vi "FA OffsetForces View.vi"(11 "Model in":refnum<class "Model.lvclass">) -> ()   [LabVIEW 2016, in "M1M3SupportEUI_Views.lvlib"]
uses:
  M1M3SupportEUI_Views.lvlib
  Model/Model.lvclass
  M1M3 Support Events/M1M3 Support Events.lvclass/M1M3 Support Events.ctl
  SALLV_m1m3/DataTypes/command_ApplyOffsetForces.ctl
  SALLV_m1m3/DataTypes/command_ClearOffsetForces.ctl
  M1M3 Support Events/M1M3 Support Events.lvclass
  EUI Events/EUI Events.lvclass
  SALLV_m1m3/SALLV_m1m3.lvlib
panel:
  in  "Z441":sgl
  in  "Z440":sgl
  in  "Z443":sgl
  in  "Z442":sgl
  in  "Z401":sgl
  in  "Z431":sgl
  in  "Z430":sgl
  in  "Z439":sgl
  in  "Z438":sgl
  in  "Z437":sgl
  in  "Z436":sgl
  in  "Z435":sgl
  in  "Z434":sgl
  in  "Z433":sgl
  in  "Z432":sgl
  in  "Z421":sgl
  in  "Z420":sgl
  in  "Z429":sgl
  in  "Z428":sgl
  in  "Z427":sgl
  in  "Z426":sgl
  in  "Z425":sgl
  in  "Z424":sgl
  in  "Z423":sgl
  in  "Z422":sgl
  in  "Z411":sgl
  in  "Z410":sgl
  in  "Z419":sgl
  in  "Z418":sgl
  in  "Z417":sgl
  in  "Z416":sgl
  in  "Z415":sgl
  in  "Z414":sgl
  in  "Z413":sgl
  in  "Z412":sgl
  in  "Z409":sgl
  in  "Z408":sgl
  in  "Z407":sgl
  in  "Z406":sgl
  in  "Z405":sgl
  in  "Z404":sgl
  in  "Z403":sgl
  in  "Z402":sgl
  in  "Z341":sgl
  in  "Z340":sgl
  in  "Z343":sgl
  in  "Z342":sgl
  in  "Z301":sgl
  in  "Z331":sgl
  in  "Z330":sgl
  in  "Z339":sgl
  in  "Z338":sgl
  in  "Z337":sgl
  in  "Z336":sgl
  in  "Z335":sgl
  in  "Z334":sgl
  in  "Z333":sgl
  in  "Z332":sgl
  in  "Z321":sgl
  in  "Z320":sgl
  in  "Z329":sgl
  in  "Z328":sgl
  in  "Z327":sgl
  in  "Z326":sgl
  in  "Z325":sgl
  in  "Z324":sgl
  in  "Z323":sgl
  in  "Z322":sgl
  in  "Z311":sgl
  in  "Z310":sgl
  in  "Z319":sgl
  in  "Z318":sgl
  in  "Z317":sgl
  in  "Z316":sgl
  in  "Z315":sgl
  in  "Z314":sgl
  in  "Z313":sgl
  in  "Z312":sgl
  in  "Z309":sgl
  in  "Z308":sgl
  in  "Z307":sgl
  in  "Z306":sgl
  in  "Z305":sgl
  in  "Z304":sgl
  in  "Z303":sgl
  in  "Z302":sgl
  in  "Z241":sgl
  in  "Z240":sgl
  in  "Z243":sgl
  in  "Z242":sgl
  in  "Z201":sgl
  in  "Z231":sgl
  in  "Z230":sgl
  in  "Z239":sgl
  in  "Z238":sgl
  in  "Z237":sgl
  in  "Z236":sgl
  in  "Z235":sgl
  in  "Z234":sgl
  in  "Z233":sgl
  in  "Z232":sgl
  in  "Z221":sgl
  in  "Z220":sgl
  in  "Z229":sgl
  in  "Z228":sgl
  in  "Z227":sgl
  in  "Z226":sgl
  in  "Z225":sgl
  in  "Z224":sgl
  in  "Z223":sgl
  in  "Z222":sgl
  in  "Z211":sgl
  in  "Z210":sgl
  in  "Z219":sgl
  in  "Z218":sgl
  in  "Z217":sgl
  in  "Z216":sgl
  in  "Z215":sgl
  in  "Z214":sgl
  in  "Z213":sgl
  in  "Z212":sgl
  in  "Z209":sgl
  in  "Z208":sgl
  in  "Z207":sgl
  in  "Z206":sgl
  in  "Z205":sgl
  in  "Z204":sgl
  in  "Z203":sgl
  in  "Z202":sgl
  in  "Y430":sgl
  in  "Y438":sgl
  in  "Y437":sgl
  in  "Y434":sgl
  in  "Y433":sgl
  in  "Y432":sgl
  in  "Y421":sgl
  in  "Y420":sgl
  in  "Y429":sgl
  in  "Y427":sgl
  in  "Y424":sgl
  in  "Y423":sgl
  in  "Y422":sgl
  in  "Y411":sgl
  in  "Y410":sgl
  in  "Y418":sgl
  in  "Y417":sgl
  in  "Y416":sgl
  in  "Y415":sgl
  in  "Y414":sgl
  in  "Y409":sgl
  in  "Y408":sgl
  in  "Y230":sgl
  in  "Y238":sgl
  in  "Y237":sgl
  in  "Y234":sgl
  in  "Y233":sgl
  in  "Y232":sgl
  in  "Y221":sgl
  in  "Y220":sgl
  in  "Y229":sgl
  in  "Y227":sgl
  in  "Y224":sgl
  in  "Y223":sgl
  in  "Y222":sgl
  in  "Y211":sgl
  in  "Y210":sgl
  in  "Y218":sgl
  in  "Y217":sgl
  in  "Y216":sgl
  in  "Y215":sgl
  in  "Y214":sgl
  in  "Y209":sgl
  in  "Y208":sgl
  in  "Y330":sgl
  in  "Y338":sgl
  in  "Y337":sgl
  in  "Y334":sgl
  in  "Y333":sgl
  in  "Y332":sgl
  in  "Y321":sgl
  in  "Y320":sgl
  in  "Y329":sgl
  in  "Y327":sgl
  in  "Y326":sgl
  in  "Y324":sgl
  in  "Y323":sgl
  in  "Y322":sgl
  in  "Y311":sgl
  in  "Y310":sgl
  in  "Y318":sgl
  in  "Y317":sgl
  in  "Y316":sgl
  in  "Y315":sgl
  in  "Y314":sgl
  in  "Y313":sgl
  in  "Y309":sgl
  in  "Y308":sgl
  in  "Y305":sgl
  in  "Y304":sgl
  in  "Y303":sgl
  in  "Y302":sgl
  in  "Z141":sgl
  in  "Z140":sgl
  in  "Z143":sgl
  in  "Z142":sgl
  in  "Z101":sgl
  in  "Z131":sgl
  in  "Z130":sgl
  in  "Z139":sgl
  in  "Z138":sgl
  in  "Z137":sgl
  in  "Z136":sgl
  in  "Z135":sgl
  in  "Z134":sgl
  in  "Z133":sgl
  in  "Z132":sgl
  in  "Z121":sgl
  in  "Z120":sgl
  in  "Z129":sgl
  in  "Z128":sgl
  in  "Z127":sgl
  in  "Z126":sgl
  in  "Z125":sgl
  in  "Z124":sgl
  in  "Z123":sgl
  in  "Z122":sgl
  in  "Z111":sgl
  in  "Z110":sgl
  in  "Z119":sgl
  in  "Z118":sgl
  in  "Z117":sgl
  in  "Z116":sgl
  in  "Z115":sgl
  in  "Z114":sgl
  in  "Z113":sgl
  in  "Z112":sgl
  in  "Z109":sgl
  in  "Z108":sgl
  in  "Z107":sgl
  in  "Z106":sgl
  in  "Z105":sgl
  in  "Z104":sgl
  in  "Z103":sgl
  in  "Z102":sgl
  in  "Y130":sgl
  in  "Y138":sgl
  in  "Y137":sgl
  in  "Y134":sgl
  in  "Y133":sgl
  in  "Y132":sgl
  in  "Y121":sgl
  in  "Y120":sgl
  in  "Y129":sgl
  in  "Y127":sgl
  in  "Y126":sgl
  in  "Y124":sgl
  in  "Y123":sgl
  in  "Y122":sgl
  in  "Y111":sgl
  in  "Y110":sgl
  in  "Y118":sgl
  in  "Y117":sgl
  in  "Y116":sgl
  in  "Y115":sgl
  in  "Y114":sgl
  in  "Y113":sgl
  in  "Y109":sgl
  in  "Y108":sgl
  in  "Y105":sgl
  in  "Y104":sgl
  in  "Y103":sgl
  in  "ClearForcesButton":bool
  in  "ApplyForcesButton":bool
  in  "Y102":sgl
  in  "X435":sgl
  in  "X428":sgl
  in  "X412":sgl
  in  "X335":sgl
  in  "X328":sgl
  in  "X312":sgl
  in  "X235":sgl
  in  "X228":sgl
  in  "X212":sgl
  in  "X135":sgl
  in  "X128":sgl
  in  "X112":sgl
  # "Force Actuator\nApply Forces"
  # "Y"
  # "Z"
  # "0"
  # "1"
  # "2"
  # "3"
  # "4"
  # "5"
  # "6"
  # "7"
  # "8"
  # "9"
  # "0"
  # "1"
  # "2"
  # "3"
  # "4"
  # "5"
  # "6"
  # "7"
  # "8"
  # "9"
  # "100"
  # "100"
  # "X"
  # "110"
  # "110"
  # "112"
  # "120"
  # "120"
  # "128"
  # "130"
  # "130"
  # "135"
  # "140"
  # "140"
  # "212"
  # "200"
  # "200"
  # "228"
  # "210"
  # "210"
  # "235"
  # "220"
  # "220"
  # "312"
  # "230"
  # "230"
  # "328"
  # "240"
  # "240"
  # "335"
  # "300"
  # "300"
  # "412"
  # "310"
  # "310"
  # "428"
  # "320"
  # "320"
  # "435"
  # "330"
  # "330"
  # "340"
  # "340"
  # "400"
  # "400"
  # "410"
  # "410"
  # "420"
  # "420"
  # "430"
  # "430"
  # "440"
  # "440"
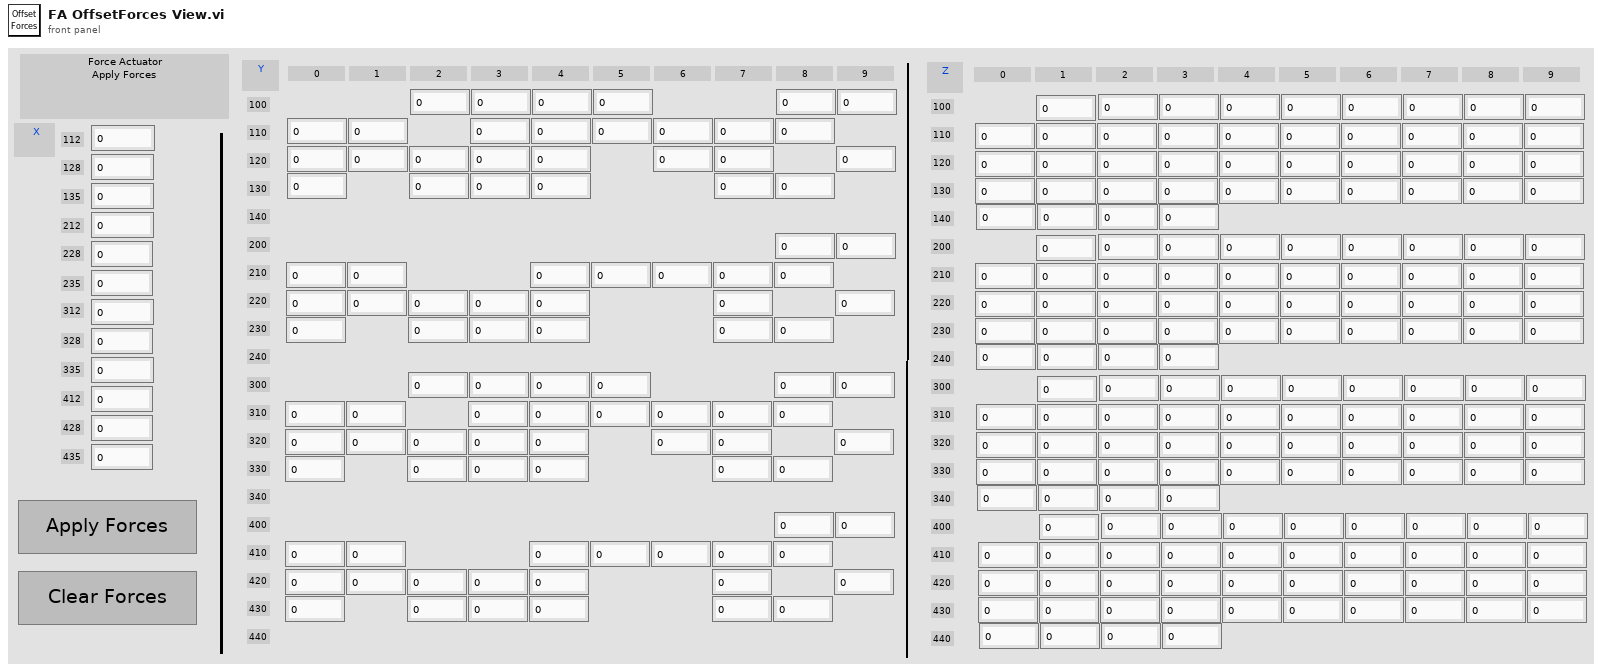
[diagram p1: front panel]
types:
  T1 = typedef "M1M3SupportEUI_TypeDefs.lvlib/M1M3 Support Events.ctl" = cluster{"Inclinometer  Data":refnum<user-event>, "IMS Data":refnum<user-event>, "FA Status":refnum<user-event>, "SAL Connected":refnum<user-event>, "Accelerometer Data":refnum<user-event>, "OuterLoop Data":refnum<user-event>, "ErrorCode Event":refnum<user-event>, "InterlockStatus Event":refnum<user-event>, "InterlockWarning Event":refnum<user-event>, "Gyro Data":refnum<user-event>, "HP Actuator Info Event":refnum<user-event>, " FA Info Event":refnum<user-event>, "HP Monitor Info Event":refnum<user-event>, "FA Data":refnum<user-event>, "HP Actuator data":refnum<user-event>, "HP Monitor data":refnum<user-event>, "Air Supply Status Event":refnum<user-event>, "Air Supply Warning Event":refnum<user-event>, "Power Data":refnum<user-event>, "PID Data":refnum<user-event>, "PID Info Event":refnum<user-event>, "Power Status Event":refnum<user-event>, "Power Supply Status Event":refnum<user-event>, "Power Warning Event":refnum<user-event>, "Summary State Event":refnum<user-event>, "Detailed State Event":refnum<user-event>}
  T2 = enum16{"", "DetailedState_DetailedStates_DisabledState", "DetailedState_DetailedStates_EnabledState", "DetailedState_DetailedStates_FaultState", "DetailedState_DetailedStates_OfflineState", "DetailedState_DetailedStates_StandbyState", "DetailedState_DetailedStates_ParkedState", "DetailedState_DetailedStates_RaisingState", "DetailedState_DetailedStates_ActiveState", "DetailedState_DetailedStates_LoweringState", "DetailedState_DetailedStates_EngineeringState", "DetailedState_DetailedStates_ParkedEngineeringState", "DetailedState_DetailedStates_RaisingEngineeringState", "DetailedState_DetailedStates_ActiveEngineeringState", "DetailedState_DetailedStates_LoweringEngineeringState", "DetailedState_DetailedStates_LoweringFaultState", "DetailedState_DetailedStates_ProfileHardpointCorrectionState"}
  T3 = typedef "SALLV_m1m3.lvlib/command_ApplyOffsetForces.ctl" = cluster{"XForces[12]":sgl[], "YForces[100]":sgl[], "ZForces[156]":sgl[]}
  T4 = typedef "SALLV_m1m3.lvlib/command_ClearOffsetForces.ctl" = cluster{"ClearOffsetForces":bool}
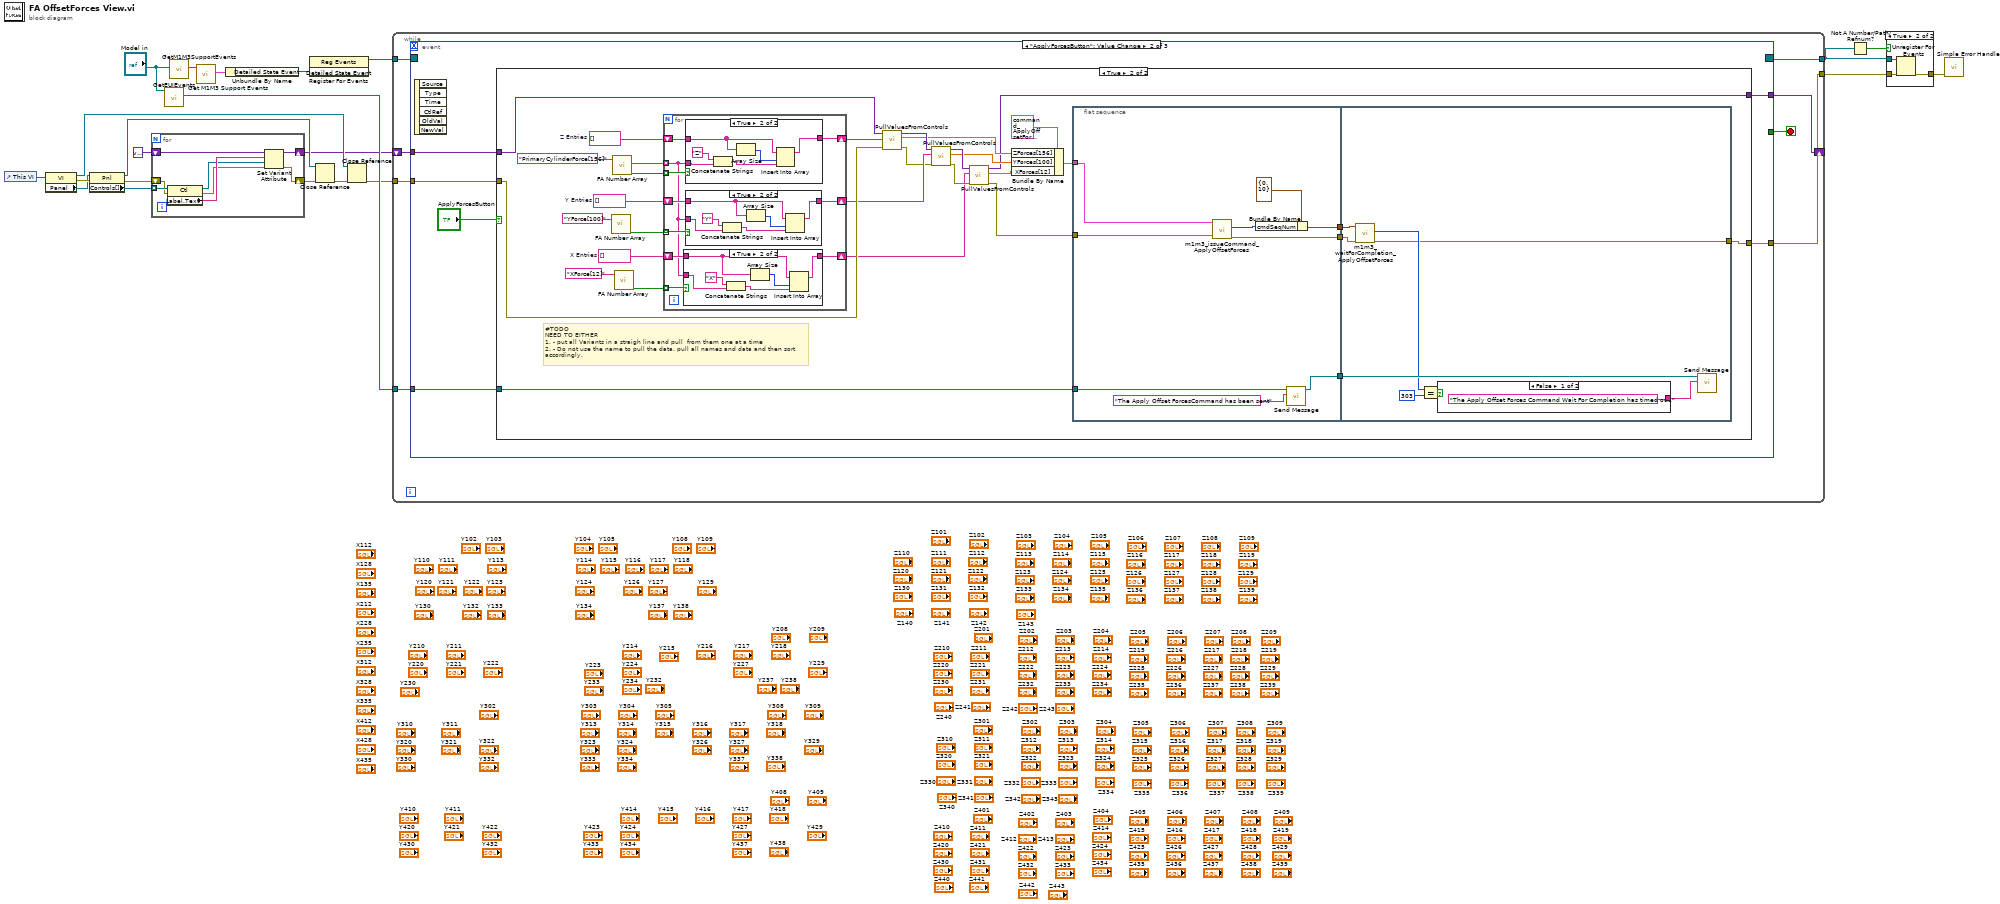
[diagram p0: block diagram]
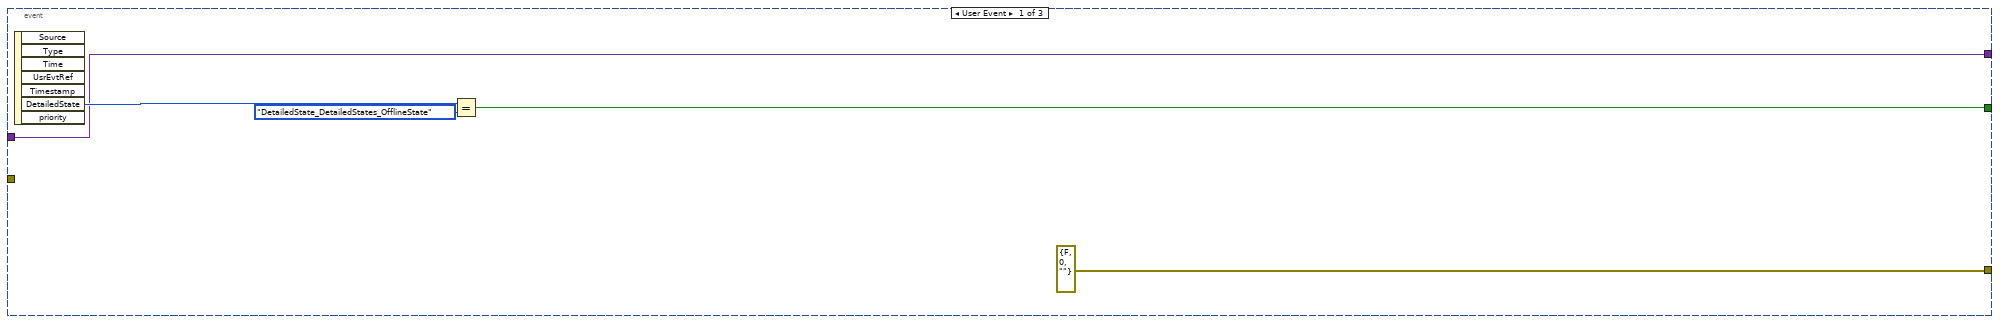
[diagram p2: hidden frame]
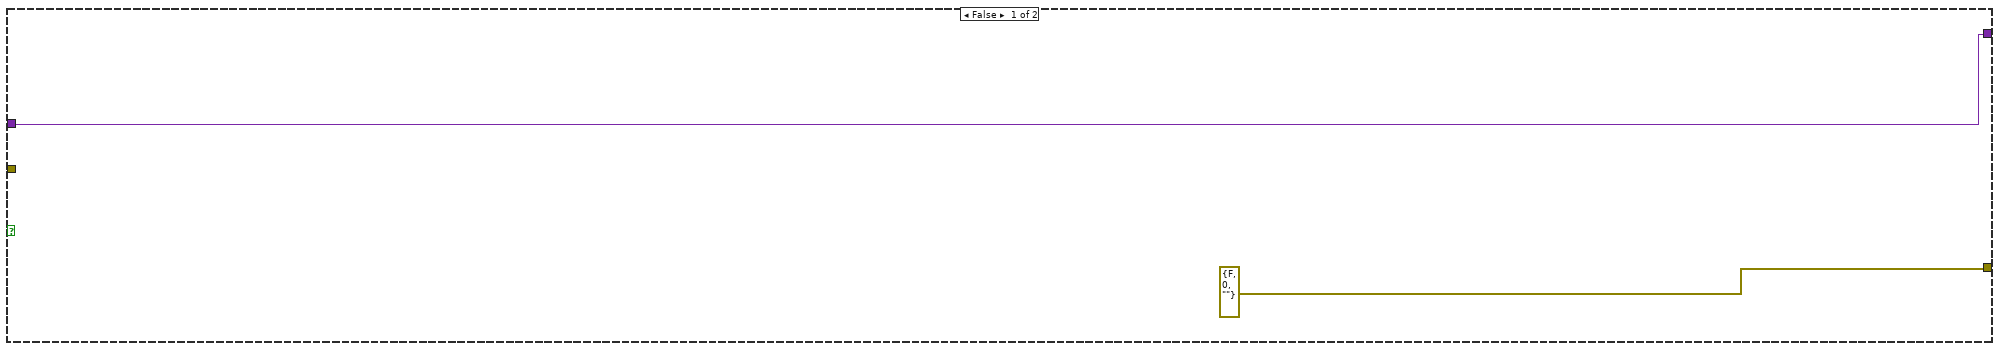
[diagram p3: hidden frame]
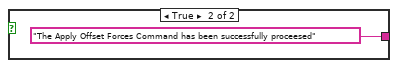
[diagram p4: hidden frame]
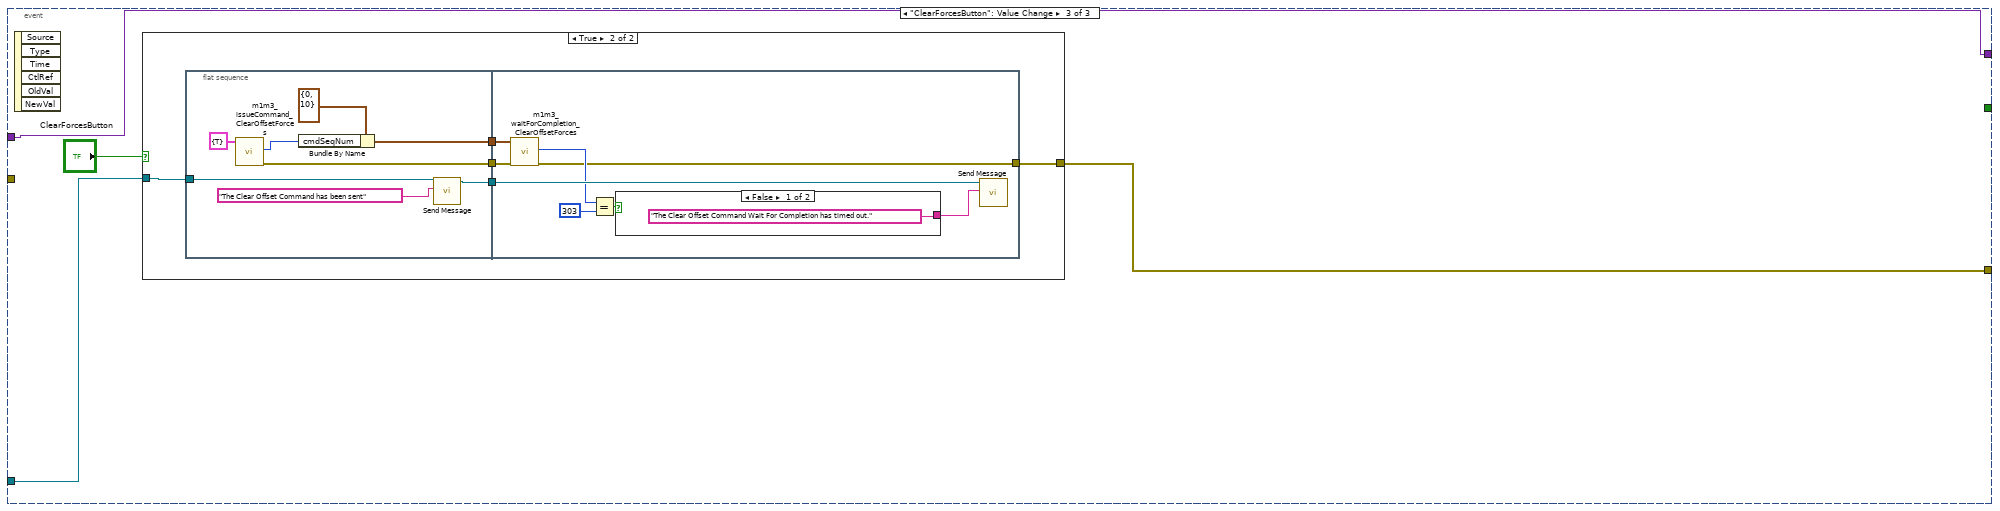
[diagram p8: hidden frame]
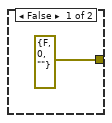
[diagram p9: hidden frame]
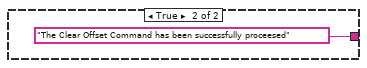
[diagram p10: hidden frame]
diagram:
  n1 = control-ref of="This VI"() -> (w12:refnum<vi>)
  n2 = property class="VI"(reference=w12) -> (reference out=w3:refnum<vi>, error out=w11:errorcluster, "Panel"=w10:refnum<vi>)  [unwired: 1 in]
  n3 = property class="Pnl"(reference=w10, error in=w11) -> (reference out=w4:refnum<vi>, error out=w7:errorcluster, "Controls[]"=w9:refnum<vi>[])
  n4 = for {
    tunnel: w9 -> [w30] mode=indexing
    shift-right: [w26] -> w2
    shift-left: variant -> [w29]
    shift-right: [w23] -> w5
    shift-left: w7 -> [w25]
    n5 = property class="Ctl"(reference=w30, error in=w25) -> (reference out=w27:refnum<vi>, error out=w24:errorcluster, "Label.Text"=w28:string)
    n6 = Set Variant Attribute(Variant=w29, name=w28, value=w27, error in=w24) -> (Variant out=w26:variant, error out=w23:errorcluster)  [unwired: 1 out]
  }
  n7 = call "GetEUIEvents.vi"("Model in"="Model in") -> ("EUI Events out"=w13:refnum<class "EUI Events.lvclass">)  [unwired: 8 in, 2 out]
  n8 = call "GetM1M3SupportEvents.vi"("Model in"="Model in") -> ("M1M3 Support Events out"=w21:refnum<class "M1M3 Support Events.lvclass">)  [unwired: 8 in, 2 out]
  n9 = call "Get M1M3 Support Events.vi"("M1M3 Support Events in"=w21) -> ("M1M3 Support Events"=w20:T1)  [unwired: 9 in, 1 out]
  n10 = Unbundle By Name(w20) -> ("Detailed State Event"=w22:refnum<user-event>)
  n11 = register-events(w22) -> (reference out=w19:refnum<event-registration>)  [unwired: 2 in, 1 out]
  n12 = Close Reference(reference=w4, error in (no error)=w5) -> (error out=w6:errorcluster)
  n13 = Close Reference(reference=w3, error in (no error)=w6) -> (error out=w1:errorcluster)
  n14 = while {
    tunnel: w19 -> [w38]
    tunnel: [w37] -> w16
    tunnel: [w34] -> w15
    tunnel: w13 -> [w35]
    tunnel: w1 -> [w32]
    shift-right: [w31] -> _
    shift-left: w2 -> [w33]
    stop <- w36 stop-if-true
    n15 = event shown="[1] \"ApplyForcesButton\": Value Change" {
      selector: w38 -> [_ _ _]
      dyn-events: [_ _ _] -> w37
      timeout: _ -> [_ _ _]
      tunnel: [w41 _ _] -> w36
      tunnel: w35 -> [_ w48 w135]
      tunnel: [errorcluster {"status"=FALSE, "code"=0, "source"=""} ("error constant") w47 w134] -> w34
      tunnel: w33 -> [w39 w46 w133]
      tunnel: w32 -> [_ w45 _]
      tunnel: [w39 w44 w133] -> w31
      event User Event {
        n16 = event-data() -> ("DetailedState"=w42:T2)  [unwired: 1 in, 6 out]
        n17 = Equal?(x=w42, y=T2."DetailedState_DetailedStates_OfflineState") -> (x = y?=w41:bool)
      }
      event "ApplyForcesButton": Value Change {
        n18 = event-data() -> ()  [unwired: 1 in, 6 out]
        n19 = case shown="True" "ApplyForcesButton" {
          tunnel: w48 -> [_ w72]
          tunnel: [errorcluster {"status"=FALSE, "code"=0, "source"=""} ("error constant") w66] -> w47
          tunnel: w46 -> [w50 w64]
          tunnel: w45 -> [_ w63]
          tunnel: [w50 w52] -> w44
          frame False {
          }
          frame True {
            w73 = string[] []  # X Entries
            w74 = string[] []  # Y Entries
            w75 = string[] []  # Z Entries
            # "#TODO\nNEED TO EITHER\n1. - put all Variants in a straigh line and pull  from them one at a time\n2. - Do not use the name to pull the data, pull all names and data and then sort accordingly."
            n20 = call "FA Number Array.vi"("Data Type"="YForce[100]") -> ("On/Off Array"=w77:bool[])  [unwired: 8 in, 2 out]
            n21 = call "FA Number Array.vi"("Data Type"="PrimaryCylinderForce[156]") -> ("On/Off Array"=w80:bool[], "FA Number String Array"=w81:string[])  [unwired: 8 in, 1 out]
            n22 = call "FA Number Array.vi"("Data Type"="XForce[12]") -> ("On/Off Array"=w76:bool[])  [unwired: 8 in, 2 out]
            n23 = for {
              tunnel: w81 -> [w102] mode=indexing
              tunnel: w80 -> [w111] mode=indexing
              tunnel: w77 -> [w108] mode=indexing
              tunnel: w76 -> [w105] mode=indexing
              shift-right: [w109] -> w65
              shift-left: w75 -> [w110]
              shift-right: [w106] -> w62
              shift-left: w74 -> [w107]
              shift-right: [w103] -> w58
              shift-left: w73 -> [w104]
              n24 = case shown="True" w105 {
                tunnel: w104 -> [w112 w115]
                tunnel: [w112 w114] -> w103
                tunnel: w102 -> [_ w113]
                frame False {
                }
                frame True {
                  n25 = Concatenate Strings("X" ("string"), w113) -> (w116:string)
                  n26 = Array Size(array=w115) -> (size(s)=w117:i32)
                  n27 = Insert Into Array(array=w115, index=w117, new element=w116) -> (w114:string[])
                }
              }
              n28 = case shown="True" w111 {
                tunnel: w102 -> [_ w131]
                tunnel: w110 -> [w126 w130]
                tunnel: [w126 w127] -> w109
                frame False {
                }
                frame True {
                  n29 = Concatenate Strings("Z" ("string"), w131) -> (w128:string)
                  n30 = Array Size(array=w130) -> (size(s)=w129:i32)
                  n31 = Insert Into Array(array=w130, index=w129, new element=w128) -> (w127:string[])
                }
              }
              n32 = case shown="True" w108 {
                tunnel: w107 -> [w119 w122]
                tunnel: w102 -> [_ w121]
                tunnel: [w119 w120] -> w106
                frame False {
                }
                frame True {
                  n33 = Concatenate Strings("Y" ("string"), w121) -> (w125:string)
                  n34 = Array Size(array=w122) -> (size(s)=w124:i32)
                  n35 = Insert Into Array(array=w122, index=w124, new element=w125) -> (w120:string[])
                }
              }
            }
            n36 = call "PullValuesFromControls.vi"("error in (no error)"=w63, "ControlNameArray"=w65, "Variant In"=w64) -> ("error out"=w60:errorcluster, "ControlValuesArray"=w54:sgl[], "Variant out"=w61:variant)  [unwired: 6 in]
            n37 = call "PullValuesFromControls.vi"("error in (no error)"=w60, "ControlNameArray"=w62, "Variant In"=w61) -> ("error out"=w59:errorcluster, "ControlValuesArray"=w55:sgl[], "Variant out"=w57:variant)  [unwired: 6 in]
            n38 = call "PullValuesFromControls.vi"("error in (no error)"=w59, "ControlNameArray"=w58, "Variant In"=w57) -> ("error out"=w53:errorcluster, "ControlValuesArray"=w56:sgl[], "Variant out"=w52:variant)  [unwired: 6 in]
            n39 = Bundle By Name(cluster=T3 {"XForces[12]"=[0.0, 0.0, 0.0, 0.0, 0.0, 0.0, 0.0, 0.0, 0.0, 0.0, 0.0, 0.0], "YForces[100]"=[0.0, 0.0, 0.0, 0.0, 0.0, 0.0, 0.0, 0.0, 0.0, 0.0, 0.0, 0.0, 0.0, 0.0, 0.0, 0.0, 0.0, 0.0, 0.0, 0.0, 0.0, 0.0, 0.0, 0.0, 0.0, 0.0, 0.0, 0.0, 0.0, 0.0, 0.0, 0.0, 0.0, 0.0, 0.0, 0.0, 0.0, 0.0, 0.0, 0.0, 0.0, 0.0, 0.0, 0.0, 0.0, 0.0, 0.0, 0.0, 0.0, 0.0, 0.0, 0.0, 0.0, 0.0, 0.0, 0.0, 0.0, 0.0, 0.0, 0.0, 0.0, 0.0, 0.0, 0.0, 0.0, 0.0, 0.0, 0.0, 0.0, 0.0, 0.0, 0.0, 0.0, 0.0, 0.0, 0.0, 0.0, 0.0, 0.0, 0.0, 0.0, 0.0, 0.0, 0.0, 0.0, 0.0, 0.0, 0.0, 0.0, 0.0, 0.0, 0.0, 0.0, 0.0, 0.0, 0.0, 0.0, 0.0, 0.0, 0.0], "ZForces[156]"=[0.0, 0.0, 0.0, 0.0, 0.0, 0.0, 0.0, 0.0, 0.0, 0.0, 0.0, 0.0, 0.0, 0.0, 0.0, 0.0, 0.0, 0.0, 0.0, 0.0, 0.0, 0.0, 0.0, 0.0, 0.0, 0.0, 0.0, 0.0, 0.0, 0.0, 0.0, 0.0, 0.0, 0.0, 0.0, 0.0, 0.0, 0.0, 0.0, 0.0, 0.0, 0.0, 0.0, 0.0, 0.0, 0.0, 0.0, 0.0, 0.0, 0.0, 0.0, 0.0, 0.0, 0.0, 0.0, 0.0, 0.0, 0.0, 0.0, 0.0, 0.0, 0.0, 0.0, 0.0, 0.0, 0.0, 0.0, 0.0, 0.0, 0.0, 0.0, 0.0, 0.0, 0.0, 0.0, 0.0, 0.0, 0.0, 0.0, 0.0, 0.0, 0.0, 0.0, 0.0, 0.0, 0.0, 0.0, 0.0, 0.0, 0.0, 0.0, 0.0, 0.0, 0.0, 0.0, 0.0, 0.0, 0.0, 0.0, 0.0, 0.0, 0.0, 0.0, 0.0, 0.0, 0.0, 0.0, 0.0, 0.0, 0.0, 0.0, 0.0, 0.0, 0.0, 0.0, 0.0, 0.0, 0.0, 0.0, 0.0, 0.0, 0.0, 0.0, 0.0, 0.0, 0.0, 0.0, 0.0, 0.0, 0.0, 0.0, 0.0, 0.0, 0.0, 0.0, 0.0, 0.0, 0.0, 0.0, 0.0, 0.0, 0.0, 0.0, 0.0, 0.0, 0.0, 0.0, 0.0, 0.0, 0.0, 0.0, 0.0, 0.0, 0.0, 0.0, 0.0]} ("command_ApplyOffsetForces_Ctl"), "ZForces[156]"=w54, "YForces[100]"=w55, "XForces[12]"=w56) -> (w69:T3)
            n40 = flat-sequence {
              tunnel: w72 -> [w91]
              tunnel: [w89] -> w71
              tunnel: w69 -> [w88]
              tunnel: w53 -> [w87]
              tunnel: [w84] -> w68
              tunnel: [w83] -> w67
              tunnel: w71 -> [w96]
              tunnel: w68 -> [w95]
              tunnel: w67 -> [w94]
              tunnel: [w92] -> w66
              frame #0 {
                n41 = call "m1m3_issueCommand_ApplyOffsetForces.vi"("error in (no error)"=w87, "command_ApplyOffsetForces_Ctl"=w88) -> ("error out"=w84:errorcluster, "function return"=w85:i32)  [unwired: 7 in, 1 out]
                n42 = Bundle By Name(cluster=cluster{"cmdSeqNum":i32, "timeout":u32} {"cmdSeqNum"=0, "timeout"=10} ("waitComplete_Ctl"), "cmdSeqNum"=w85) -> (w83:cluster{"cmdSeqNum":i32, "timeout":u32})
                n43 = call "Send Message.vi"("Message"="The Apply Offset ForcesCommand has been sent", "EUI Events in"=w91) -> ("EUI Events out"=w89:refnum<class "EUI Events.lvclass">)  [unwired: 8 in, 1 out]
              }
              frame #1 {
                n44 = call "m1m3_waitForCompletion_ApplyOffsetForces.vi"("error in (no error)"=w95, "waitComplete_Ctl"=w94) -> ("error out"=w92:errorcluster, "function return"=w93:i32)  [unwired: 7 in, 1 out]
                n45 = Equal?(x=w93, y=303) -> (x = y?=w98:bool)
                n46 = case shown="False" w98 {
                  tunnel: ["The Apply Offset Forces Command Wait For Completion has timed out." ("Message") "The Apply Offset Forces Command has been successfully proceesed" ("Message")] -> w97
                  frame False {
                  }
                  frame True {
                  }
                }
                n47 = call "Send Message.vi"("Message"=w97, "EUI Events in"=w96) -> ()  [unwired: 8 in, 2 out]
              }
            }
          }
        }
      }
      event "ClearForcesButton": Value Change {
        n48 = event-data() -> ()  [unwired: 1 in, 6 out]
        n49 = case shown="True" "ClearForcesButton" {
          tunnel: w135 -> [_ w142]
          tunnel: [errorcluster {"status"=FALSE, "code"=0, "source"=""} ("error constant") w138] -> w134
          frame False {
          }
          frame True {
            n50 = flat-sequence {
              tunnel: w142 -> [w149]
              tunnel: [w145] -> w141
              tunnel: [w144] -> w140
              tunnel: [w143] -> w139
              tunnel: w141 -> [w158]
              tunnel: w140 -> [w157]
              tunnel: w139 -> [w153]
              tunnel: [w151] -> w138
              frame #0 {
                n51 = call "m1m3_issueCommand_ClearOffsetForces.vi"("command_ClearOffsetForces_Ctl"=T4 {"ClearOffsetForces"=TRUE}) -> ("error out"=w145:errorcluster, "function return"=w146:i32)  [unwired: 8 in, 1 out]
                n52 = Bundle By Name(cluster=cluster{"cmdSeqNum":i32, "timeout":u32} {"cmdSeqNum"=0, "timeout"=10} ("waitComplete_Ctl"), "cmdSeqNum"=w146) -> (w144:cluster{"cmdSeqNum":i32, "timeout":u32})
                n53 = call "Send Message.vi"("Message"="The Clear Offset Command has been sent", "EUI Events in"=w149) -> ("EUI Events out"=w143:refnum<class "EUI Events.lvclass">)  [unwired: 8 in, 1 out]
              }
              frame #1 {
                n54 = call "m1m3_waitForCompletion_ClearOffsetForces.vi"("error in (no error)"=w158, "waitComplete_Ctl"=w157) -> ("error out"=w151:errorcluster, "function return"=w152:i32)  [unwired: 7 in, 1 out]
                n55 = Equal?(x=w152, y=303) -> (x = y?=w155:bool)
                n56 = case shown="False" w155 {
                  tunnel: ["The Clear Offset Command Wait For Completion has timed out." ("Message") "The Clear Offset Command has been successfully proceesed" ("Message")] -> w156
                  frame False {
                  }
                  frame True {
                  }
                }
                n57 = call "Send Message.vi"("Message"=w156, "EUI Events in"=w153) -> ()  [unwired: 8 in, 2 out]
              }
            }
          }
        }
      }
    }
  }
  n58 = Not A Number/Path/Refnum?(number/path/refnum=w16) -> (NaN/Path/Refnum?=w17:bool)
  n59 = case shown="True" w17 {
    tunnel: w16 -> [_ w164]
    tunnel: w15 -> [w161 w163]
    tunnel: [w161 w162] -> w18
    frame False {
    }
    frame True {
      n60 = Unregister For Events(event registration refnum=w164, error in=w163) -> (error out=w162:errorcluster)
    }
  }
  n61 = call <vilib>:"Simple Error Handler.vi"("error in (no error)"=w18) -> ()  [unwired: 4 in, 5 out]
